vi "jobbatchData.vi"() -> ()   [LabVIEW 2012]
uses:
  <vilib>/addons/database/Auxilliary.llb/DB Tools Cursor Type.ctl
  <vilib>/addons/database/Connection.llb/DB Tools Open Connec (Path).vi
  <vilib>/addons/database/Connection.llb/Conn Execute.vi
  <vilib>/addons/database/Recordset.llb/Rec Fetch Recordset Data (R).vi
  <vilib>/addons/database/Recordset.llb/Rec Destroy - Connection.vi
  <vilib>/addons/database/NI_Database_API.lvlib
panel:
  out "recordset data":variant[][](array[variant])
  in  "Lotno":string
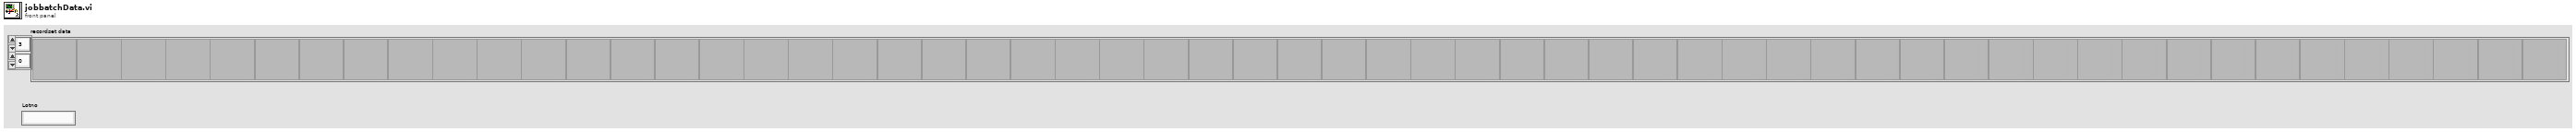
[diagram p1: front panel]
types:
  T1 = typedef "NI_Database_API.lvlib/DB Tools Cursor Type.ctl" = enum16{"forward-only", "keyset", "dynamic", "static"}
  T2 = typedef "NI_Database_API.lvlib/Conn ObjectReference.ctl" = refnum<k1>
  T3 = typedef "NI_Database_API.lvlib/Rec ObjectReference.ctl" = refnum<k1>
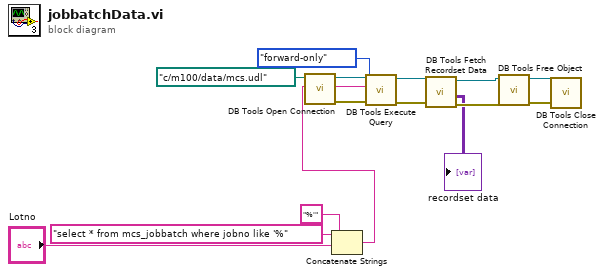
[diagram p0: block diagram]
diagram:
  n1 = call-poly <vilib>:"DB Tools Open Connection.vi"("connection information"=path "c:/m100/data/mcs.udl") -> ("error out"=w9:errorcluster, "connection reference"=w12:T2)  [unwired: 7 in]
  n2 = Concatenate Strings("select * from mcs_jobbatch where jobno like '%" ("string"), "Lotno", "%'" ("string")) -> (w2:string)
  n3 = call-poly <vilib>:"DB Tools Execute Query.vi"("error in (no error)"=w9, "cursor type"=DB_Tools_Cursor_Type."forward-only", "SQL query"=w2, "connection reference"=w12) -> ("error out"=w8:errorcluster, "recordset reference"=w11:T3)  [unwired: 4 in]
  n4 = call-poly <vilib>:"DB Tools Fetch Recordset Data.vi"("error in (no error)"=w8, "recordset reference"=w11) -> ("error out"=w7:errorcluster, "recordset data"=→"recordset data":variant[][], "recordset reference out"=w10:T3)  [unwired: 3 in]
  n5 = call-poly <vilib>:"DB Tools Free Object.vi"("error in (no error)"=w7, "recordset reference"=w10) -> ("error out"=w14:errorcluster, "connection reference"=w13:T2)  [unwired: 8 in]
  n6 = call <vilib>:"DB Tools Close Connection.vi"("error in (no error)"=w14, "connection reference"=w13) -> ()  [unwired: 5 in, 1 out]
